vi "TreeNode Get Tree.vi"(8 "error in (no error)":errorcluster, 11 "TreeNode DVR in":refnum<data-value>) -> (0 "error out":errorcluster, 2 "Tree out":refnum<data-value>, 3 "TreeNode DVR out":refnum<data-value>)   [LabVIEW 2010, in "MDSplus.lvlib"]
doc: "Get Data for this node."
uses:
  <vilib>/MDSplus/Library/MDSplus.lvlib
  <vilib>/MDSplus/Classes/Data_Class/TreeNode_Class/TreeNode.lvclass
  <vilib>/MDSplus/Classes/Tree_Class/Tree.lvclass
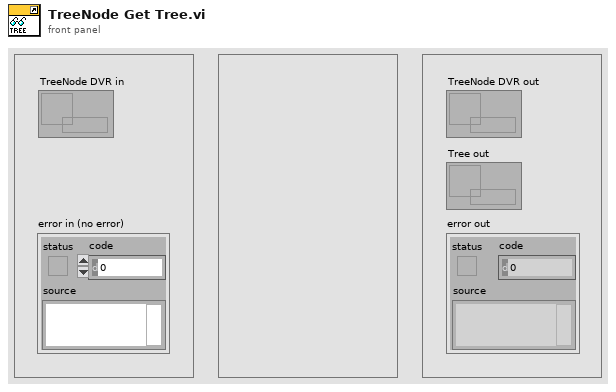
[diagram p1: front panel]
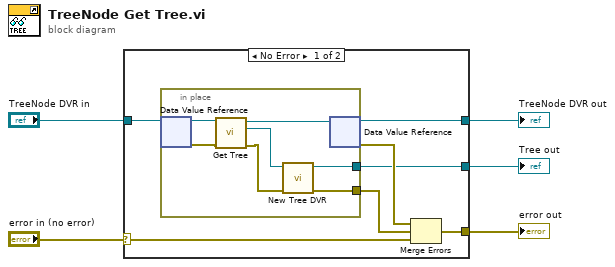
[diagram p0: block diagram]
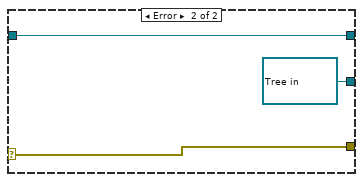
[diagram p2: hidden frame]
diagram:
  n1 = case shown="No Error" "error in (no error)" {
    selector: "error in (no error)" -> [w11 w22]
    tunnel: "TreeNode DVR in" -> [w12 w21]
    tunnel: [w8 w22] -> w5
    tunnel: [w9 w21] -> w2
    tunnel: [w6 refnum<data-value> refnum ("Tree DVR out")] -> w1
    frame No Error {
      n2 = in-place {
        in-place-border: [w13] -> w7
        in-place-border: [w14] -> w6
        n3 = in-place-dvr #1(w12) -> (w19:refnum<class "TreeNode.lvclass">, w18:errorcluster)
        n4 = call-dynamic "Get Tree.vi"("error in (no error)"=w18, "TreeNode in"=w19) -> ("error out"=w17:errorcluster, "Tree out"=w15:refnum<class "Tree.lvclass">, "TreeNode out"=w16:refnum<class "TreeNode.lvclass">)  [unwired: 7 in]
        n5 = call <vilib>:"New Tree DVR.vi"("error in (no error)"=w17, "Tree in"=w15) -> ("error out"=w13:errorcluster, "Tree DVR out"=w14:refnum<data-value>)  [unwired: 8 in]
        n6 = in-place-dvr #1(w16) -> (w9:refnum<data-value>, w10:errorcluster)
      }
      n7 = Merge Errors(w10, w7, w11) -> (w8:errorcluster)
    }
    frame Error {
    }
  }
  "error out" <- w5
  "TreeNode DVR out" <- w2
  "Tree out" <- w1
